vi "Rename.vi"(8 "error in (no error)":errorcluster, 10 "New Name":string, 11 "Name":string) -> (0 "error out":errorcluster)   [LabVIEW 2017, in "TimerEngine.lvlib" / "TimerEngine.lvclass"]
uses:
  TimerEngine.lvclass
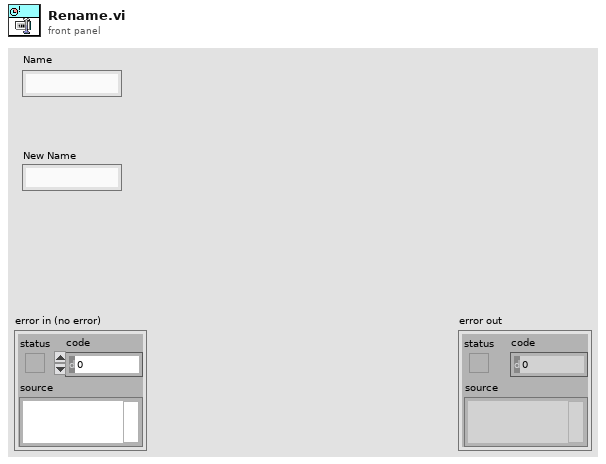
[diagram p1: front panel]
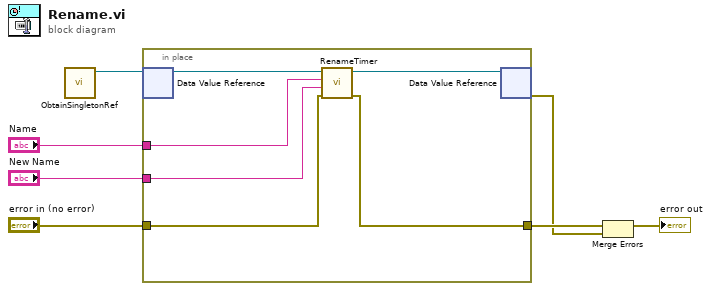
[diagram p0: block diagram]
diagram:
  n1 = call "ObtainSingletonRef.vi"() -> ("data value reference"=w7:refnum<data-value>)  [unwired: 9 in, 2 out]
  n2 = in-place {
    in-place-border: [w10] -> w6
    in-place-border: "error in (no error)" -> [w11]
    in-place-border: "Name" -> [w9]
    in-place-border: "New Name" -> [w8]
    n3 = in-place-dvr #1(w7) -> (w13:refnum<class "TimerEngine.lvclass">)  [unwired: 1 out]
    n4 = call "RenameTimer.vi"("error in (no error)"=w11, "New Name"=w8, "Name"=w9, "TimerEngine in"=w13) -> ("error out"=w10:errorcluster, "TimerEngine out"=w12:refnum<class "TimerEngine.lvclass">)  [unwired: 6 in]
    n5 = in-place-dvr #1(w12) -> (w3:errorcluster)  [unwired: 1 out]
  }
  n6 = Merge Errors(w6, w3) -> (→"error out":errorcluster)
